vi "assignTreeTag.vi"(6 "reservedTreeTags[]":string[](array[string]), 8 "error in (no error)":errorcluster, 10 "TreeCtl*":refnum<vi>, 11 "xceDataNode in":refnum<class "xceDataNode.lvclass">) -> (0 "error out":errorcluster, 3 "xceDataNode out":refnum<class "xceDataNode.lvclass">)   [LabVIEW 2013, in "xceDataNode.lvclass"]
doc: "Assigns a unique tree tag to the xceDataNode. The treeTag is the universal way to identify this node from the rest. Recursive if you wish to assign a treeTag to this node, and all of its subnodes."
uses:
  xceDataNode/xceDataNode.lvclass
  xceNode/xceNode.lvclass
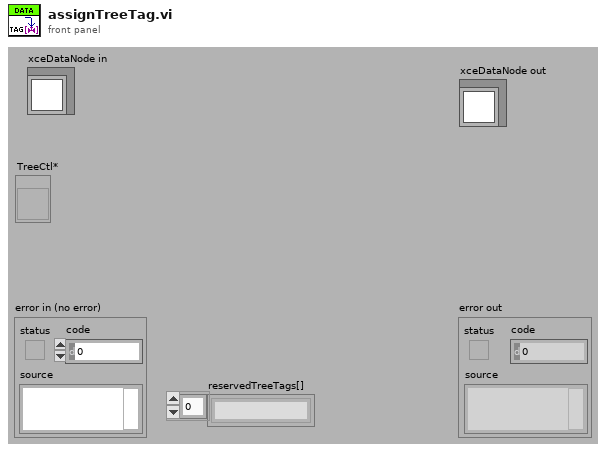
[diagram p1: front panel]
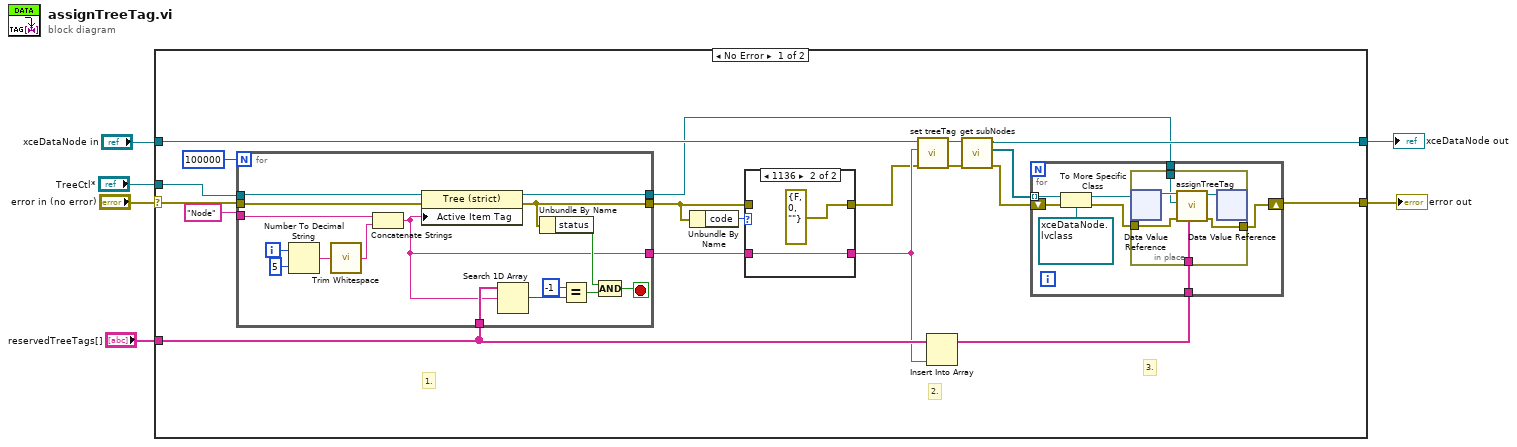
[diagram p0: block diagram]
diagram:
  n1 = case shown="No Error" "error in (no error)" {
    selector: "error in (no error)" -> [w23 w60]
    tunnel: [w19 w60] -> w1
    tunnel: [w10 w59] -> w2
    tunnel: "xceDataNode in" -> [w14 w59]
    tunnel: "reservedTreeTags[]" -> [w18 _]
    tunnel: "TreeCtl*" -> [w17 _]
    frame No Error {
      # "3."
      # "2."
      # "1."
      n2 = for {
        N: 100000 -> [_]
        tunnel: "Node" -> [w53]
        tunnel: w17 -> [w58]
        tunnel: [w45] -> w20
        tunnel: w23 -> [w52]
        tunnel: [w51] -> w21
        tunnel: w18 -> [w50]
        tunnel: [w43] -> w7
        i -> [w57]
        stop <- w44 stop-if-true
        n3 = Number To Decimal String(number=w57, width (-)=i16 5) -> (decimal integer string=w55:string)
        n4 = call <vilib>:"Trim Whitespace.vi"("string"=w55) -> ("trimmed string"=w54:string)  [unwired: 1 in]
        n5 = Concatenate Strings(w53, w54) -> (w45:string)
        n6 = property class="Tree (strict)"(reference=w58, error in=w52, "Active Item Tag"=w45) -> (reference out=w43:refnum<vi>, error out=w51:errorcluster)
        n7 = Search 1D Array(1D array=w50, element=w45) -> (index of element=w49:i32)  [unwired: 1 in]
        n8 = Unbundle By Name(w51) -> ("status"=w46:bool)
        n9 = Equal?(x=-1, y=w49) -> (x = y?=w47:bool)
        n10 = Compound Arithmetic op=AND(w46, w47) -> (w44:bool)
      }
      n11 = Unbundle By Name(w21) -> ("code"=w22:i32)
      n12 = case shown="1136" w22 {
        tunnel: w21 -> [w40 _]
        tunnel: [w40 errorcluster {"status"=FALSE, "code"=0, "source"=""} ("error out")] -> w9
        tunnel: w20 -> [_ w41]
        tunnel: [_ w41] -> w13
        frame Default {
        }
        frame 1136 {
        }
      }
      n13 = call "set treeTag.vi"("error in (no error)"=w9, "treeTag"=w13, "xceNode in"=w14) -> ("error out"=w16:errorcluster, "xceNode out"=w15:refnum<class "xceDataNode.lvclass">)  [unwired: 7 in]
      n14 = Insert Into Array(array=w18, new element=w13) -> (w11:string[])  [unwired: 1 in]
      n15 = call "get subNodes.vi"("error in (no error)"=w16, "xceNode in"=w15) -> ("error out"=w8:errorcluster, "subNodes[]*"=w12:refnum<data-value>[], "xceNode out"=w10:refnum<class "xceDataNode.lvclass">)  [unwired: 7 in]
      n16 = for {
        tunnel: w12 -> [w33] mode=indexing
        shift-right: [w27] -> w19
        shift-left: w8 -> [w32]
        tunnel: w11 -> [w30]
        tunnel: w7 -> [w26]
        n17 = To More Specific Class(target class=refnum<data-value> refnum ("data value reference"), reference=w33, error in=w32) -> (specific class reference=w31:refnum<data-value>, error out=w28:errorcluster)
        n18 = in-place {
          in-place-border: w30 -> [w39]
          in-place-border: w28 -> [w36]
          in-place-border: [w35] -> w27
          in-place-border: w26 -> [w34]
          n19 = in-place-dvr #1(w31) -> (w38:refnum<class "xceDataNode.lvclass">)  [unwired: 1 out]
          n20 = call "assignTreeTag.vi"("reservedTreeTags[]"=w39, "error in (no error)"=w36, "TreeCtl*"=w34, "xceDataNode in"=w38) -> ("error out"=w35:errorcluster, "xceDataNode out"=w37:refnum<class "xceDataNode.lvclass">)  [unwired: 6 in]
          n21 = in-place-dvr #1(w37) -> ()  [unwired: 2 out]
        }
      }
    }
    frame Error {
    }
  }
  "error out" <- w1
  "xceDataNode out" <- w2
